vi "start.vi"(8 "error in (no error)":errorcluster, 10 "start":bool, 11 "AtomChipHWC in":refnum<class "AtomChipHWC.lvclass">) -> (0 "error out":errorcluster, 2 "started":bool, 3 "AtomChipHWC out":refnum<class "AtomChipHWC.lvclass">)   [LabVIEW 2011, in "Hardware.lvlib" / "HWControllers.lvlib" / "AtomChipHWC.lvclass"]
doc: "Start running an experiment. I.e. Start all hardware."
uses:
  AtomChipHWC.lvclass
  AtomChipHWC.lvclass/AtomChipHWC.ctl
  HardwareConfiguration/HWConfiguration.lvclass
  Channels/Digital/DigitalOutput.lvclass
  Channels/VoltOutput/AnalogOutput.lvclass
  Channels/DDSOutput/Generic/DDSOutput.lvclass
  Tools/Filing/FileNeologist/FileNeologist.lvclass
  HWController.lvclass
  Tools/Filing.lvlib
panel:
  out "time to start":dbl
  # "not used here"
  # "not used here"
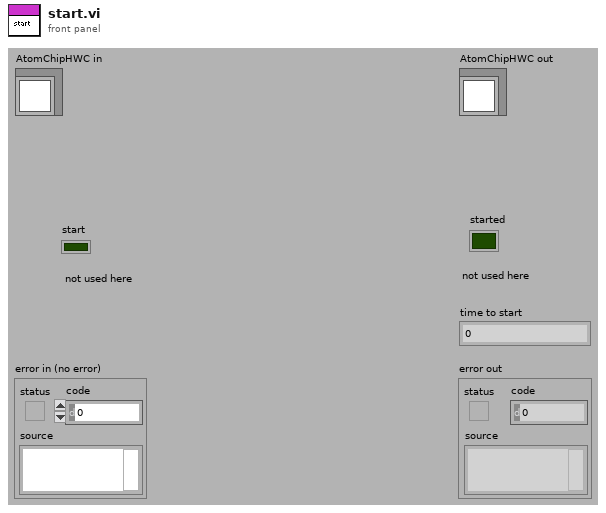
[diagram p1: front panel]
types:
  T1 = enum16{"Ready", "Compiling", "Configured", "Running", "Stopping", "Unresolved Error"}
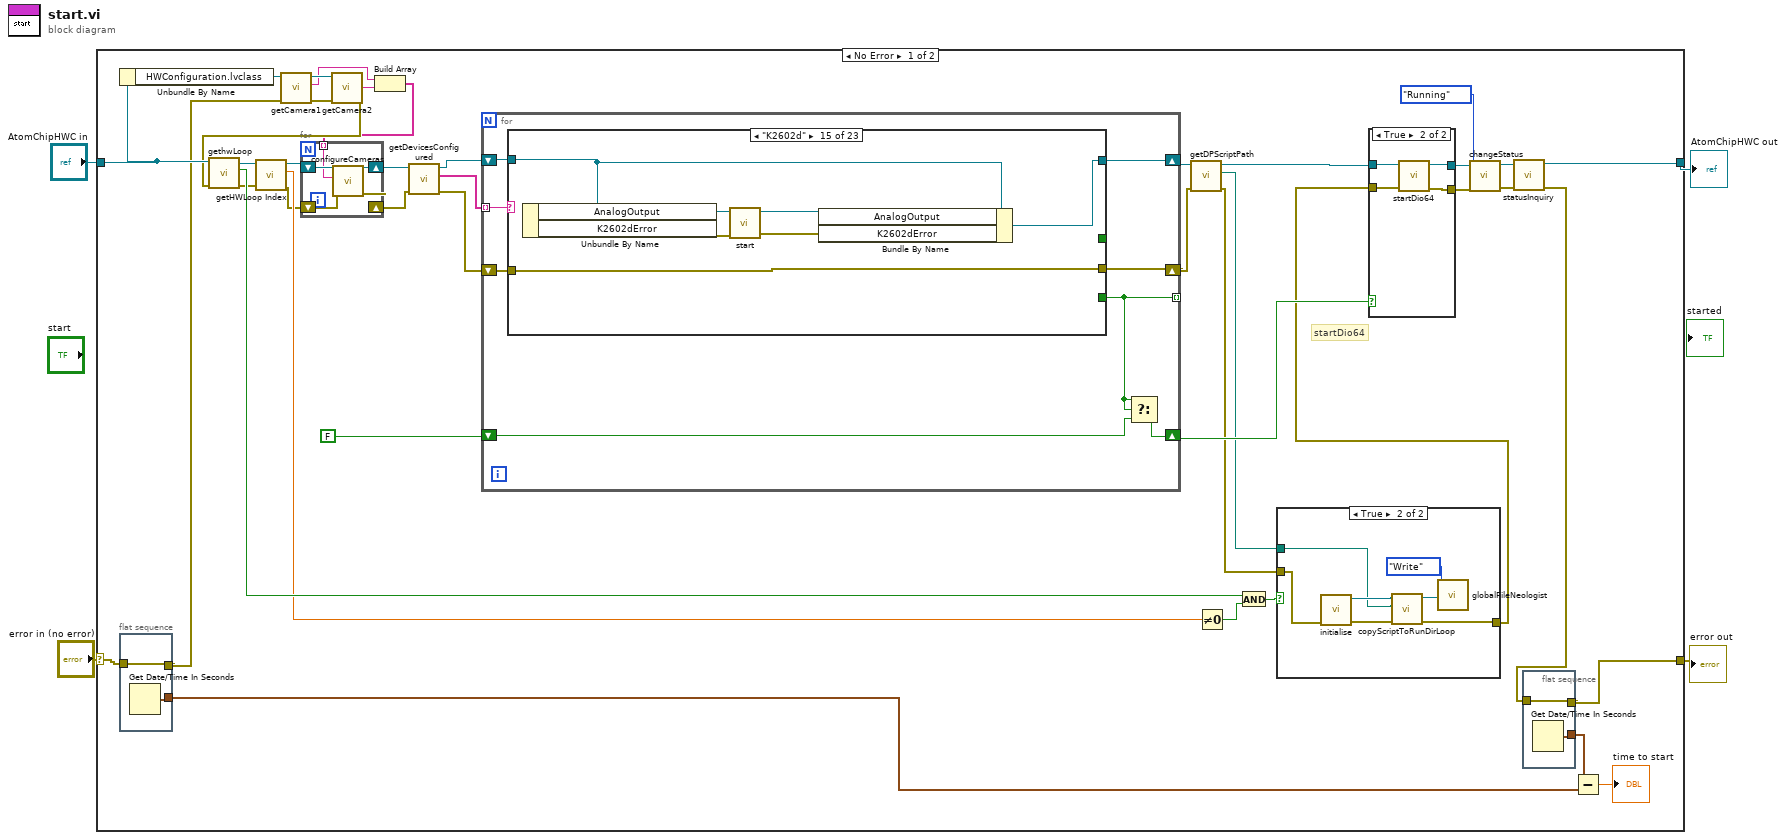
[diagram p0: block diagram]
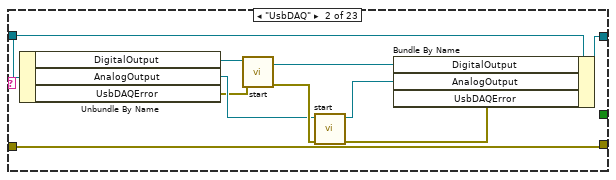
[diagram p5: hidden frame]
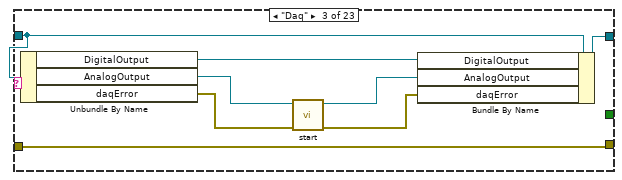
[diagram p6: hidden frame]
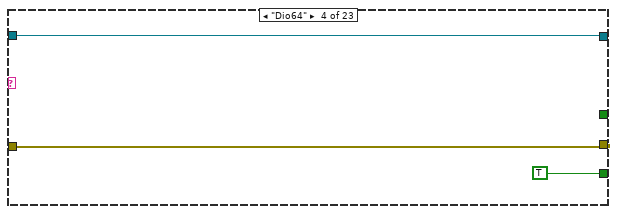
[diagram p7: hidden frame]
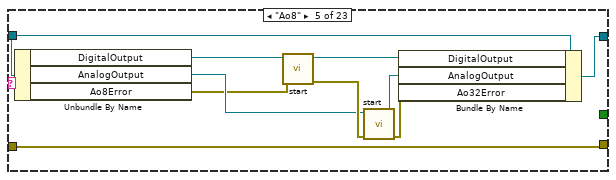
[diagram p8: hidden frame]
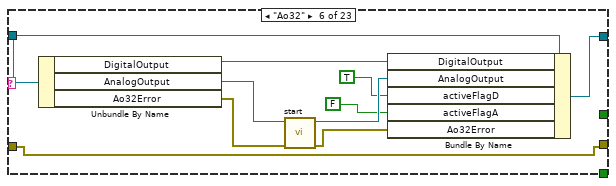
[diagram p9: hidden frame]
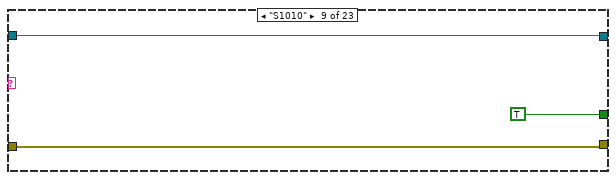
[diagram p12: hidden frame]
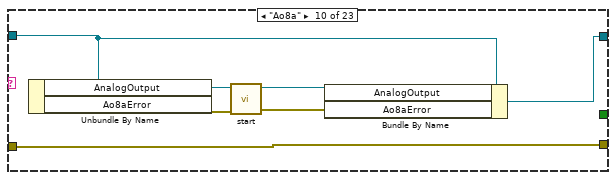
[diagram p13: hidden frame]
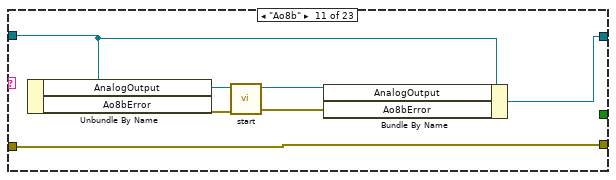
[diagram p14: hidden frame]
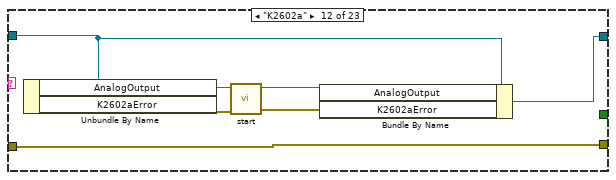
[diagram p15: hidden frame]
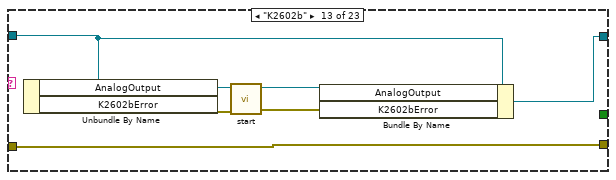
[diagram p16: hidden frame]
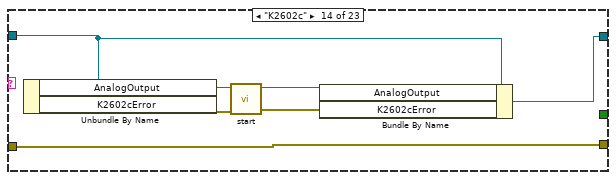
[diagram p17: hidden frame]
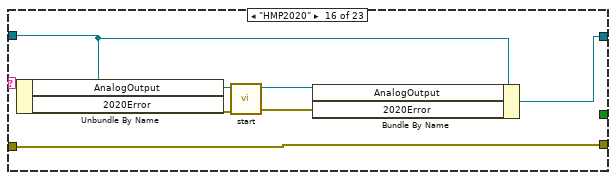
[diagram p18: hidden frame]
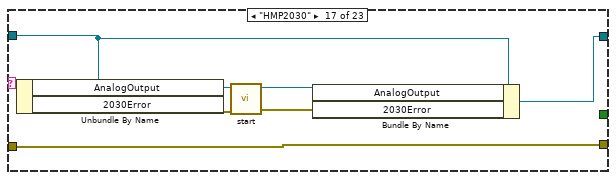
[diagram p19: hidden frame]
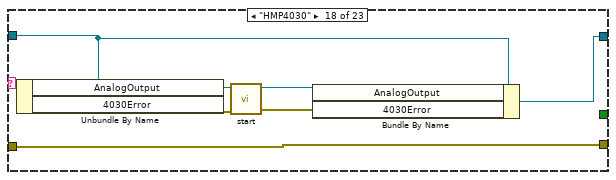
[diagram p20: hidden frame]
diagram:
  n1 = case shown="No Error" "error in (no error)" {
    selector: "error in (no error)" -> [w26 w224]
    tunnel: [w23 w224] -> w3
    tunnel: [w46 w225] -> w1
    tunnel: "AtomChipHWC in" -> [w45 w225]
    frame No Error {
      # "startDio64"
      n2 = Unbundle By Name(w45) -> ("HWConfiguration.lvclass"=w39:refnum<class "HWConfiguration.lvclass">)
      n3 = flat-sequence {
        tunnel: [w55] -> w25
        tunnel: w26 -> [w55]
        tunnel: [w54] -> w21
        frame #0 {
          n4 = Get Date/Time In Seconds() -> (seconds since 1Jan1904=w54:timestamp)
        }
      }
      n5 = call-dynamic "getCamera1.vi"("error in (no error)"=w25, "HWConfiguration.lvclass in"=w39) -> ("error out"=w18:errorcluster, "camera1"=w16:string, "HWConfiguration.lvclass out"=w19:refnum<class "HWConfiguration.lvclass">)  [unwired: 7 in]
      n6 = call-dynamic "getCamera2.vi"("error in (no error)"=w18, "HWConfiguration.lvclass in"=w19) -> ("error out"=w17:errorcluster, "camera2"=w15:string)  [unwired: 7 in, 1 out]
      n7 = call "gethwLoop.vi"("error in (no error)"=w17, "HWController in"=w45) -> ("error out"=w36:errorcluster, "hwLoop?"=w38:bool, "HWController out"=w37:refnum<class "AtomChipHWC.lvclass">)  [unwired: 7 in]
      n8 = call "getHWLoop Index.vi"("error in (no error)"=w36, "HWController in"=w37) -> ("error out"=w10:errorcluster, "HWLoop Index"=w35:dbl, "HWController out"=w11:refnum<class "AtomChipHWC.lvclass">)  [unwired: 7 in]
      n9 = Build Array(w16, w15) -> (w14:string[])
      n10 = for {
        shift-right: [w48] -> w9
        shift-left: w11 -> [w51]
        shift-right: [w47] -> w6
        shift-left: w10 -> [w50]
        tunnel: w14 -> [w49] mode=indexing
        n11 = call "configureCameras.vi"("error in (no error)"=w50, "deviceName"=w49, "AtomChipHWC in"=w51) -> ("error out"=w47:errorcluster, "AtomChipHWC out"=w48:refnum<class "AtomChipHWC.lvclass">)  [unwired: 7 in]
      }
      n12 = call "getDevicesConfigured.vi"("error in (no error)"=w6, "HWController.lvclass in"=w9) -> ("error out"=w5:errorcluster, "devicesConfigured"=w7:string[], "HWController.lvclass out"=w8:refnum<class "AtomChipHWC.lvclass">)  [unwired: 7 in]
      n13 = for {
        tunnel: w7 -> [w76] mode=indexing
        shift-right: [w74] -> w32
        shift-left: w8 -> [w77]
        shift-right: [w73] -> w31
        shift-left: w5 -> [w75]
        tunnel: [w72] -> _ mode=indexing
        shift-right: [w70] -> w44
        shift-left: FALSE -> [w71]
        n14 = case shown="\"K2602d\"" w76 {
          selector: w76 -> [_ _ _ _ _ _ _ _ _ _ _ _ _ _ _ _ _ _ _ _ _ _ w219]
          tunnel: [w79 w88 w97 w100 w108 w120 w122 w124 w127 w133 w140 w147 w154 w161 w168 w175 w182 w189 w197 w204 w211 w218 w222] -> w74
          tunnel: [w78 w80 w90 w99 w101 w111 w121 w123 w126 w128 w135 w142 w149 w156 w163 w170 w177 w184 w191 w198 w205 w212 w221] -> w73
          tunnel: w77 -> [w79 w89 w96 w100 w109 w119 w122 w124 w127 w132 w139 w146 w153 w160 w167 w174 w181 w188 w196 w203 w210 w217 w223]
          tunnel: w75 -> [w78 w80 w90 w99 w101 w111 w121 w123 w126 w128 w135 w142 w149 w156 w163 w170 w177 w184 w191 w198 w205 w212 w220]
          tunnel: [_ _ _ TRUE _ _ _ _ _ _ _ _ _ _ _ _ _ _ _ _ _ _ _] -> w72
          tunnel: [_ _ _ _ _ _ _ _ TRUE _ _ _ _ _ _ _ _ _ _ _ _ _ _] -> _
          frame "No Hardware", Default {
          }
          frame "UsbDAQ" {
            n15 = Unbundle By Name(w89) -> ("DigitalOutput"=w86:refnum<class "DigitalOutput.lvclass">, "AnalogOutput"=w85:refnum<class "AnalogOutput.lvclass">, "UsbDAQError"=w81:errorcluster)
            n16 = call-dynamic "start.vi"("error in (no error)"=w81, "DigitalOutput in"=w86) -> ("error out"=w87:errorcluster, "DigitalOutput out"=w84:refnum<class "DigitalOutput.lvclass">)  [unwired: 8 in]
            n17 = call-dynamic "start.vi"("error in (no error)"=w87, "AnalogOutput in"=w85) -> ("error out"=w82:errorcluster, "AnalogOutput out"=w83:refnum<class "AnalogOutput.lvclass">)  [unwired: 8 in]
            n18 = Bundle By Name(cluster=w89, "DigitalOutput"=w84, "AnalogOutput"=w83, "UsbDAQError"=w82) -> (w88:refnum<class "AtomChipHWC.lvclass">)
          }
          frame "Daq" {
            n19 = Unbundle By Name(w96) -> ("DigitalOutput"=w93:refnum<class "DigitalOutput.lvclass">, "AnalogOutput"=w95:refnum<class "AnalogOutput.lvclass">, "daqError"=w92:errorcluster)
            n20 = call-dynamic "start.vi"("error in (no error)"=w92, "AnalogOutput in"=w95) -> ("error out"=w91:errorcluster, "AnalogOutput out"=w94:refnum<class "AnalogOutput.lvclass">)  [unwired: 8 in]
            n21 = Bundle By Name(cluster=w96, "DigitalOutput"=w93, "AnalogOutput"=w94, "daqError"=w91) -> (w97:refnum<class "AtomChipHWC.lvclass">)
          }
          frame "Dio64" {
          }
          frame "Ao8" {
            n22 = Unbundle By Name(w109) -> ("DigitalOutput"=w107:refnum<class "DigitalOutput.lvclass">, "AnalogOutput"=w104:refnum<class "AnalogOutput.lvclass">, "Ao8Error"=w102:errorcluster)
            n23 = call-dynamic "start.vi"("error in (no error)"=w102, "DigitalOutput in"=w107) -> ("error out"=w110:errorcluster, "DigitalOutput out"=w106:refnum<class "DigitalOutput.lvclass">)  [unwired: 8 in]
            n24 = call-dynamic "start.vi"("error in (no error)"=w110, "AnalogOutput in"=w104) -> ("error out"=w103:errorcluster, "AnalogOutput out"=w105:refnum<class "AnalogOutput.lvclass">)  [unwired: 8 in]
            n25 = Bundle By Name(cluster=w109, "DigitalOutput"=w106, "AnalogOutput"=w105, "Ao32Error"=w103) -> (w108:refnum<class "AtomChipHWC.lvclass">)
          }
          frame "Ao32" {
            n26 = Unbundle By Name(w119) -> ("DigitalOutput"=w116:refnum<class "DigitalOutput.lvclass">, "AnalogOutput"=w118:refnum<class "AnalogOutput.lvclass">, "Ao32Error"=w112:errorcluster)
            n27 = call-dynamic "start.vi"("error in (no error)"=w112, "AnalogOutput in"=w118) -> ("error out"=w113:errorcluster, "AnalogOutput out"=w117:refnum<class "AnalogOutput.lvclass">)  [unwired: 8 in]
            n28 = Bundle By Name(cluster=w119, "DigitalOutput"=w116, "AnalogOutput"=w117, "activeFlagD"=TRUE, "activeFlagA"=FALSE, "Ao32Error"=w113) -> (w120:refnum<class "AtomChipHWC.lvclass">)
          }
          frame "ICCamera" {
          }
          frame "AndorIKon" {
          }
          frame "S1010" {
          }
          frame "Ao8a" {
            n29 = Unbundle By Name(w132) -> ("AnalogOutput"=w134:refnum<class "AnalogOutput.lvclass">, "Ao8aError"=w130:errorcluster)
            n30 = call-dynamic "start.vi"("error in (no error)"=w130, "AnalogOutput in"=w134) -> ("error out"=w129:errorcluster, "AnalogOutput out"=w131:refnum<class "AnalogOutput.lvclass">)  [unwired: 8 in]
            n31 = Bundle By Name(cluster=w132, "AnalogOutput"=w131, "Ao8aError"=w129) -> (w133:refnum<class "AtomChipHWC.lvclass">)
          }
          frame "Ao8b" {
            n32 = Unbundle By Name(w139) -> ("AnalogOutput"=w141:refnum<class "AnalogOutput.lvclass">, "Ao8bError"=w137:errorcluster)
            n33 = call-dynamic "start.vi"("error in (no error)"=w137, "AnalogOutput in"=w141) -> ("error out"=w136:errorcluster, "AnalogOutput out"=w138:refnum<class "AnalogOutput.lvclass">)  [unwired: 8 in]
            n34 = Bundle By Name(cluster=w139, "AnalogOutput"=w138, "Ao8bError"=w136) -> (w140:refnum<class "AtomChipHWC.lvclass">)
          }
          frame "K2602a" {
            n35 = Unbundle By Name(w146) -> ("AnalogOutput"=w148:refnum<class "AnalogOutput.lvclass">, "K2602aError"=w144:errorcluster)
            n36 = call-dynamic "start.vi"("error in (no error)"=w144, "AnalogOutput in"=w148) -> ("error out"=w143:errorcluster, "AnalogOutput out"=w145:refnum<class "AnalogOutput.lvclass">)  [unwired: 8 in]
            n37 = Bundle By Name(cluster=w146, "AnalogOutput"=w145, "K2602aError"=w143) -> (w147:refnum<class "AtomChipHWC.lvclass">)
          }
          frame "K2602b" {
            n38 = Unbundle By Name(w153) -> ("AnalogOutput"=w155:refnum<class "AnalogOutput.lvclass">, "K2602bError"=w151:errorcluster)
            n39 = call-dynamic "start.vi"("error in (no error)"=w151, "AnalogOutput in"=w155) -> ("error out"=w150:errorcluster, "AnalogOutput out"=w152:refnum<class "AnalogOutput.lvclass">)  [unwired: 8 in]
            n40 = Bundle By Name(cluster=w153, "AnalogOutput"=w152, "K2602bError"=w150) -> (w154:refnum<class "AtomChipHWC.lvclass">)
          }
          frame "K2602c" {
            n41 = Unbundle By Name(w160) -> ("AnalogOutput"=w162:refnum<class "AnalogOutput.lvclass">, "K2602cError"=w158:errorcluster)
            n42 = call-dynamic "start.vi"("error in (no error)"=w158, "AnalogOutput in"=w162) -> ("error out"=w157:errorcluster, "AnalogOutput out"=w159:refnum<class "AnalogOutput.lvclass">)  [unwired: 8 in]
            n43 = Bundle By Name(cluster=w160, "AnalogOutput"=w159, "K2602cError"=w157) -> (w161:refnum<class "AtomChipHWC.lvclass">)
          }
          frame "K2602d" {
            n44 = Unbundle By Name(w167) -> ("AnalogOutput"=w169:refnum<class "AnalogOutput.lvclass">, "K2602dError"=w165:errorcluster)
            n45 = call-dynamic "start.vi"("error in (no error)"=w165, "AnalogOutput in"=w169) -> ("error out"=w164:errorcluster, "AnalogOutput out"=w166:refnum<class "AnalogOutput.lvclass">)  [unwired: 8 in]
            n46 = Bundle By Name(cluster=w167, "AnalogOutput"=w166, "K2602dError"=w164) -> (w168:refnum<class "AtomChipHWC.lvclass">)
          }
          frame "HMP2020" {
            n47 = Unbundle By Name(w174) -> ("AnalogOutput"=w176:refnum<class "AnalogOutput.lvclass">, "2020Error"=w172:errorcluster)
            n48 = call-dynamic "start.vi"("error in (no error)"=w172, "AnalogOutput in"=w176) -> ("error out"=w171:errorcluster, "AnalogOutput out"=w173:refnum<class "AnalogOutput.lvclass">)  [unwired: 8 in]
            n49 = Bundle By Name(cluster=w174, "AnalogOutput"=w173, "2020Error"=w171) -> (w175:refnum<class "AtomChipHWC.lvclass">)
          }
          frame "HMP2030" {
            n50 = Unbundle By Name(w181) -> ("AnalogOutput"=w183:refnum<class "AnalogOutput.lvclass">, "2030Error"=w179:errorcluster)
            n51 = call-dynamic "start.vi"("error in (no error)"=w179, "AnalogOutput in"=w183) -> ("error out"=w178:errorcluster, "AnalogOutput out"=w180:refnum<class "AnalogOutput.lvclass">)  [unwired: 8 in]
            n52 = Bundle By Name(cluster=w181, "AnalogOutput"=w180, "2030Error"=w178) -> (w182:refnum<class "AtomChipHWC.lvclass">)
          }
          frame "HMP4030" {
            n53 = Unbundle By Name(w188) -> ("AnalogOutput"=w190:refnum<class "AnalogOutput.lvclass">, "4030Error"=w186:errorcluster)
            n54 = call-dynamic "start.vi"("error in (no error)"=w186, "AnalogOutput in"=w190) -> ("error out"=w185:errorcluster, "AnalogOutput out"=w187:refnum<class "AnalogOutput.lvclass">)  [unwired: 8 in]
            n55 = Bundle By Name(cluster=w188, "AnalogOutput"=w187, "4030Error"=w185) -> (w189:refnum<class "AtomChipHWC.lvclass">)
          }
          frame "SpinCoreDDS0" {
            n56 = Unbundle By Name(w196) -> ("DDSOutput"=w195:refnum<class "DDSOutput.lvclass">, "DDS0Error"=w193:errorcluster)
            n57 = call-dynamic "start.vi"("error in (no error)"=w193, "DDSOutput in"=w195) -> ("error out"=w192:errorcluster, "DDSOutput out"=w194:refnum<class "DDSOutput.lvclass">)  [unwired: 8 in]
            n58 = Bundle By Name(cluster=w196, "DDSOutput"=w194, "DDS0Error"=w192) -> (w197:refnum<class "AtomChipHWC.lvclass">)
          }
          frame "SpinCoreDDS1" {
            n59 = Unbundle By Name(w203) -> ("DDSOutput"=w202:refnum<class "DDSOutput.lvclass">, "DDS1Error"=w200:errorcluster)
            n60 = call-dynamic "start.vi"("error in (no error)"=w200, "DDSOutput in"=w202) -> ("error out"=w199:errorcluster, "DDSOutput out"=w201:refnum<class "DDSOutput.lvclass">)  [unwired: 8 in]
            n61 = Bundle By Name(cluster=w203, "DDSOutput"=w201, "DDS1Error"=w199) -> (w204:refnum<class "AtomChipHWC.lvclass">)
          }
          frame "CQTDDS0" {
            n62 = Unbundle By Name(w210) -> ("DDSOutput"=w209:refnum<class "DDSOutput.lvclass">, "DDS0Error"=w207:errorcluster)
            n63 = call-dynamic "start.vi"("error in (no error)"=w207, "DDSOutput in"=w209) -> ("error out"=w206:errorcluster, "DDSOutput out"=w208:refnum<class "DDSOutput.lvclass">)  [unwired: 8 in]
            n64 = Bundle By Name(cluster=w210, "DDSOutput"=w208, "DDS0Error"=w206) -> (w211:refnum<class "AtomChipHWC.lvclass">)
          }
          frame "k3390" {
            n65 = Unbundle By Name(w217) -> ("DDSOutput"=w216:refnum<class "DDSOutput.lvclass">, "DDS1Error"=w214:errorcluster)
            n66 = call-dynamic "start.vi"("error in (no error)"=w214, "DDSOutput in"=w216) -> ("error out"=w213:errorcluster, "DDSOutput out"=w215:refnum<class "DDSOutput.lvclass">)  [unwired: 8 in]
            n67 = Bundle By Name(cluster=w217, "DDSOutput"=w215, "DDS1Error"=w213) -> (w218:refnum<class "AtomChipHWC.lvclass">)
          }
          frame "PixelFly", "Pixis", "ProEM" {
            n68 = call "startCamera.vi"("error in (no error)"=w220, "camera"=w219, "AtomChipHWC in"=w223) -> ("error out"=w221:errorcluster, "AtomChipHWC out"=w222:refnum<class "AtomChipHWC.lvclass">)  [unwired: 7 in]
          }
        }
        n69 = Select(t=w72, s=w72, f=w71) -> (s? t:f=w70:bool)
      }
      n70 = call "getDPScriptPath.vi"("error in (no error)"=w31, "HWController in"=w32) -> ("error out"=w29:errorcluster, "DPScriptPath"=w30:path, "HWController out"=w13:refnum<class "AtomChipHWC.lvclass">)  [unwired: 7 in]
      n71 = Not Equal To 0?(x=w35) -> (x != 0?=w34:bool)
      n72 = And(x=w38, y=w34) -> (x .and. y?=w33:bool)
      n73 = case shown="True" w33 {
        tunnel: w29 -> [w56 w62]
        tunnel: w30 -> [_ w58]
        tunnel: [w56 w60] -> w12
        frame False {
        }
        frame True {
          n74 = call "initialise.vi"("error in (no error)"=w62) -> ("error out"=w61:errorcluster, "FileNeologist out"=w59:refnum<class "FileNeologist.lvclass">)  [unwired: 9 in]
          n75 = call-dynamic "copyScriptToRunDirLoop.vi"("error in (no error)"=w61, "Path in"=w58, "FileNeologist in"=w59) -> ("error out"=w60:errorcluster, "FileNeologist out"=w57:refnum<class "FileNeologist.lvclass">)  [unwired: 6 in, 1 out]
          n76 = call "globalFileNeologist.vi"("FileNeologist in"=w57, "Action"=enum16{"Write", "Read"}."Write") -> ()  [unwired: 9 in, 1 out]
        }
      }
      n77 = case shown="True" w44 {
        tunnel: w13 -> [w65 w69]
        tunnel: [w65 w68] -> w28
        tunnel: w12 -> [w64 w67]
        tunnel: [w64 w66] -> w27
        frame False {
        }
        frame True {
          n78 = call "startDio64.vi"("error in (no error)"=w67, "AtomChipHWC in"=w69) -> ("error out"=w66:errorcluster, "AtomChipHWC out"=w68:refnum<class "AtomChipHWC.lvclass">)  [unwired: 8 in]
        }
      }
      n79 = call "changeStatus.vi"("error in (no error)"=w27, "status"=T1."Running", "HWController in"=w28) -> ("error out"=w42:errorcluster, "HWController out"=w43:refnum<class "AtomChipHWC.lvclass">)  [unwired: 7 in]
      n80 = call-dynamic "statusInquiry.vi"("error in (no error)"=w42, "HWController in"=w43) -> ("error out"=w24:errorcluster, "HWController out"=w46:refnum<class "AtomChipHWC.lvclass">)  [unwired: 8 in]
      n81 = flat-sequence {
        tunnel: [w53] -> w23
        tunnel: w24 -> [w53]
        tunnel: [w52] -> w22
        frame #0 {
          n82 = Get Date/Time In Seconds() -> (seconds since 1Jan1904=w52:timestamp)
        }
      }
      n83 = Subtract(x=w22, y=w21) -> (x-y=→"time to start":dbl)
    }
    frame Error {
    }
  }
  "error out" <- w3
  "AtomChipHWC out" <- w1
